vi "GetkA(K-182) v0.1.vi"(0 "Keithley 182 GPIB":string="2", 1 "error in":errorcluster) -> (2 "Voltage (V)":dbl=-1.943291 format="%.6f", 3 "Magnet Current (kA)":dbl=-7.773164 format="%.6f", 4 "error out":errorcluster)   [LabVIEW 2024]
panel:
  in  "Command":string="g0x"
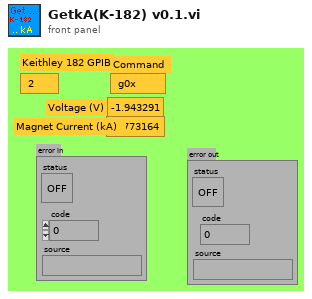
[diagram p1: front panel]
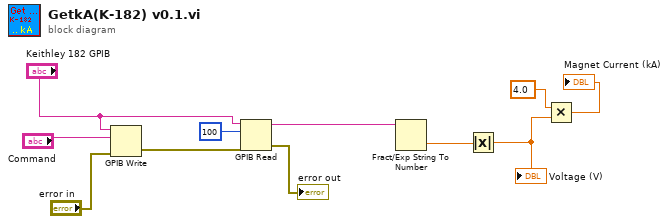
[diagram p0: block diagram]
diagram:
  n1 = GPIB Write(0:"Keithley 182 GPIB", 1:"Command", 3:"error in") -> (6:w3:errorcluster)  [unwired: 2 in, 1 out]
  n2 = GPIB Read(0:"Keithley 182 GPIB", 1:100, 3:w3) -> (5:w11:string, 7:→"error out":errorcluster)  [unwired: 2 in, 1 out]
  n3 = Fract/Exp String To Number(string=w11) -> (number=w2:dbl)  [unwired: 3 in, 1 out]
  n4 = Absolute Value(x=w2) -> (abs(x)=w1:dbl)
  "Voltage (V)" <- w1
  n5 = Multiply(x=4.0, y=w1) -> (x*y=→"Magnet Current (kA)":dbl)
